vi "Practica_2.vi"() -> ()   [LabVIEW 2020]
uses:
  <vilib>/express/express shared/transition.llb/Dynamic To Waveform Array.vi
  <vilib>/express/express signal manip/GetorSetDDTAttributes/Set DDT Attributes/SetT0.vi
  <vilib>/express/express shared/transition.llb/Waveform Array To Dynamic.vi
  <vilib>/express/express signal manip/GetorSetDDTAttributes/Set DDT Attributes/Set DDT Properties.xnode
panel:
  in  "Flush? (T)":bool=TRUE
  out "x .and. y?":bool
  out "Waveform Chart 3":dbl[](graph)
  in  "Max":dbl
  in  "Min":dbl
  out "Waveform Chart 2":dbl[](graph)
  out "Frecuencia":dbl format="%#_13g"
  out "Waveform Chart":dynamicdata(graph)
  in  "stop":bool
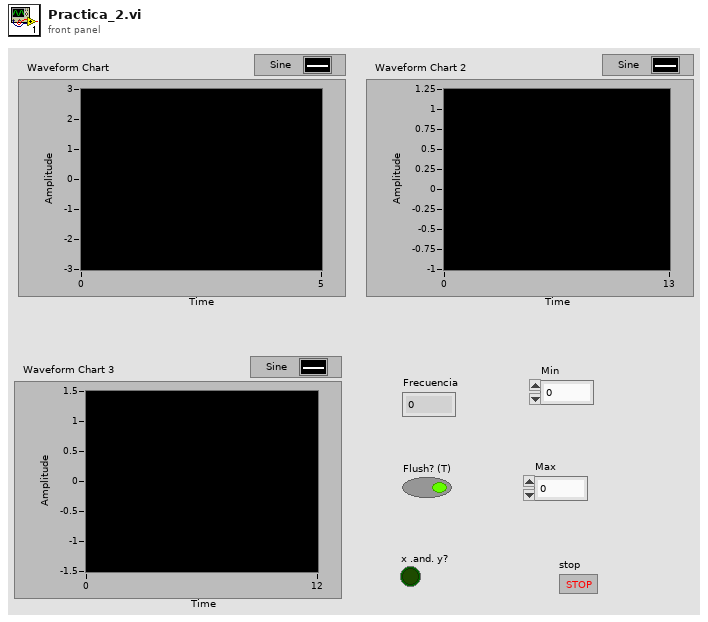
[diagram p1: front panel]
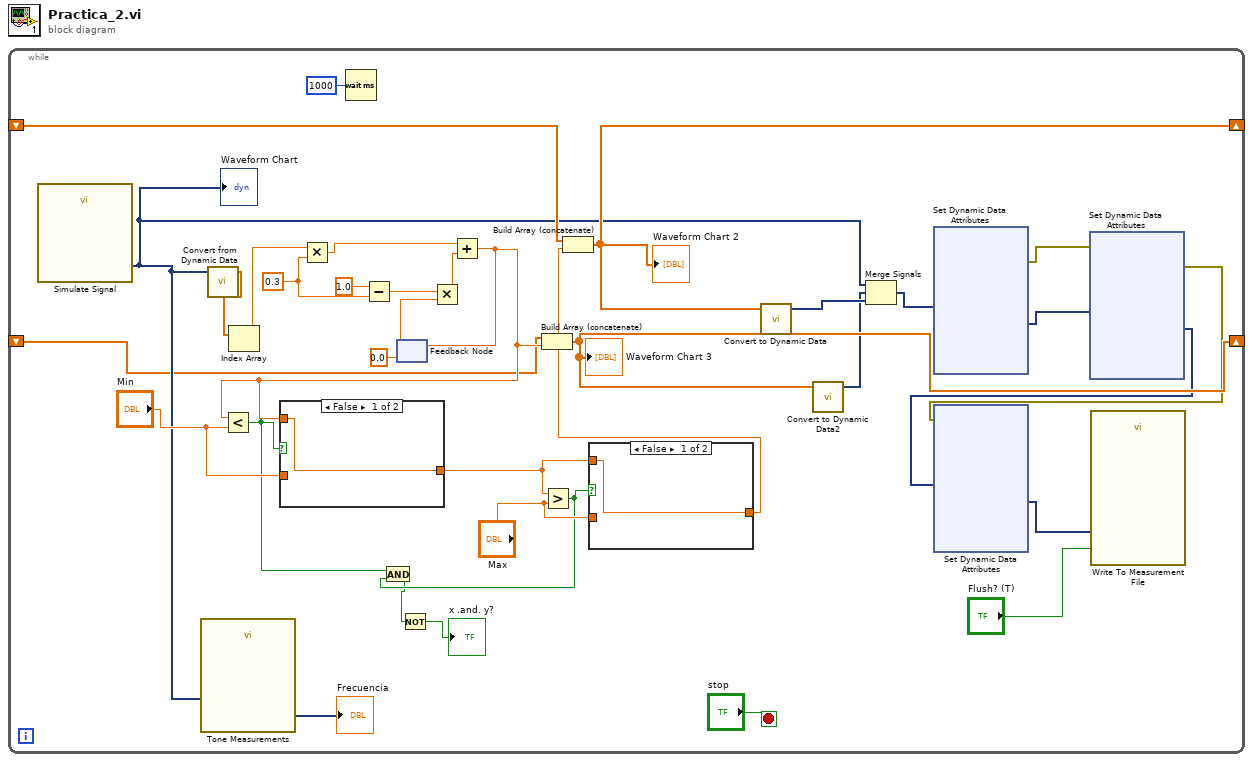
[diagram p0: block diagram]
diagram:
  n1 = while {
    shift-right: [w16] -> _
    shift-left: _ -> [w24]
    shift-right: [w13] -> _
    shift-left: _ -> [w12]
    stop <- "stop" stop-if-true
    w33 = 0.3 ("y")
    n2 = call "Simulate Signal"() -> ("Sine"=w15:dynamicdata)  [unwired: 14 in, 1 out]
    "Waveform Chart" <- w15
    n3 = call "Tone Measurements"("Signals"=w15) -> ("Frequency"=→"Frecuencia":dynamicdata)  [unwired: 9 in, 1 out]
    n4 = call "Convert from Dynamic Data"("Dynamic Data Type"=w15) -> ("Array"=w26:dbl[])  [unwired: 3 in]
    n5 = Index Array(array=w26) -> (element=w25:dbl)  [unwired: 1 in]
    n6 = Multiply(x=w25, y=w33) -> (x*y=w29:dbl)
    n7 = Wait (ms)(milliseconds to wait=u32 1000) -> ()  [unwired: 1 out]
    n8 = Subtract(x=1.0, y=w33) -> (x-y=w31:dbl)
    n9 = feedback #1(0.0) -> (w28:dbl)
    n10 = Multiply(x=w31, y=w28) -> (x*y=w30:dbl)
    n11 = Add(x=w29, y=w30) -> (x+y=w14:dbl)
    n12 = Less?(x=w14, y="Min") -> (x < y?=w18:bool)
    n13 = case shown="False" w18 {
      tunnel: "Min" -> [_ w81]
      tunnel: [w80 w81] -> w20
      tunnel: w14 -> [w80 _]
      frame False {
      }
      frame True {
      }
    }
    n14 = feedback-in #1(w14) -> ()
    n15 = Build Array (concatenate)(w12, w14) -> (w13:dbl[])
    "Waveform Chart 3" <- w13
    n16 = Greater?(x=w20, y="Max") -> (0:w17:bool)
    n17 = And(x=w18, y=w17) -> (x .and. y?=w11:bool)
    n18 = Not(x=w11) -> (.not. x?=→"x .and. y?":bool)
    n19 = case shown="False" w17 {
      tunnel: "Max" -> [_ w79]
      tunnel: [w78 w79] -> w19
      tunnel: w20 -> [w78 _]
      frame False {
      }
      frame True {
      }
    }
    n20 = Build Array (concatenate)(w24, w19) -> (w16:dbl[])
    "Waveform Chart 2" <- w16
    n21 = call "Convert to Dynamic Data"("Array"=w16) -> ("Dynamic Data Type"=w4:dynamicdata)  [unwired: 3 in]
    n22 = call "Convert to Dynamic Data2"("Array"=w13) -> ("Dynamic Data Type"=w3:dynamicdata)  [unwired: 3 in]
    n23 = Merge Signals(w15, w3, w4) -> (w5:dynamicdata)
    n24 = xnode "Set Dynamic Data Attributes"("Signals In"=w5) -> ("Signals Out"=w1:dynamicdata, "error out"=w2:errorcluster)  [unwired: 3 in]
    n25 = xnode "Set Dynamic Data Attributes"("Signals In"=w1, "error in"=w2) -> ("Signals Out"=w7:dynamicdata, "error out"=w6:errorcluster)  [unwired: 2 in]
    n26 = xnode "Set Dynamic Data Attributes"("Signals In"=w7, "error in"=w6) -> ("Signals Out"=w8:dynamicdata)  [unwired: 2 in, 1 out]
    n27 = call "Write To Measurement File"("Signals"=w8, "Flush? (T)"="Flush? (T)") -> ()  [unwired: 15 in, 3 out]
  }
